vi "ListFiles.vi"() -> ()   [LabVIEW 2010]
uses:
  EDSDK-Labview.llb/kEdsStorageType.ctl
  EDSDK-Labview.llb/EdsAccess.ctl
  EDSDK-Labview.llb/kEdsTargetImageTypes.ctl
  EDSDK-Labview.llb/kEdsImageTypes.ctl
  EDSDK-Labview.llb/EdsImageQuality.ctl
  EDSDK-Labview.llb/kEdsProperties.ctl
  EDSDK-Labview.llb/kEdsImageSrcs.ctl
panel:
  out "timing details":cluster{"FileName":string, u32, "Numeric":dbl}[](array[cluster])
  in  "Image Type":T1=4 items=["Grayscale (U8)", "Grayscale (I16)", "Grayscale (SGL)", "Complex (CSG)", "RGB (U32)", "HSL (U32)", "RGB (U64)", "Grayscale (U16)"]
  out "dt":u32
  out "current file":string
  in  "full/thumbnail":bool
  in  "stop":bool
  out "Image Out":T2(plugin-control)
  out "files":T4(array[cluster]) {"format" items=["Unknown"=0, "Jpeg"=1, "CRW"=2, "RAW"=4, "CR2"=6, "MOVwithTHM"=12, "MOVwithoutTHM"=13]}
  out "subfolders":T6(array[cluster]) {"format" items=["Unknown"=0, "Jpeg"=1, "TIFF"=7, "TIFF16"=8, "RGB"=9, "RGB16"=10, "DIB"=11]}
  out "folders":T6(array[cluster]) {"format" items=["Unknown"=0, "Jpeg"=1, "TIFF"=7, "TIFF16"=8, "RGB"=9, "RGB16"=10, "DIB"=11]}
  out "disks":T9(array[cluster]) {"kEdsStorageType" items=["Non"=0, "CF"=1, "SD"=2, "HD"=4]; "EdsAccess" items=["ReadOnly"=0, "WriteOnly"=1, "ReadWrite"=2, "Error"=4294967295]}
  out "cameras":u32
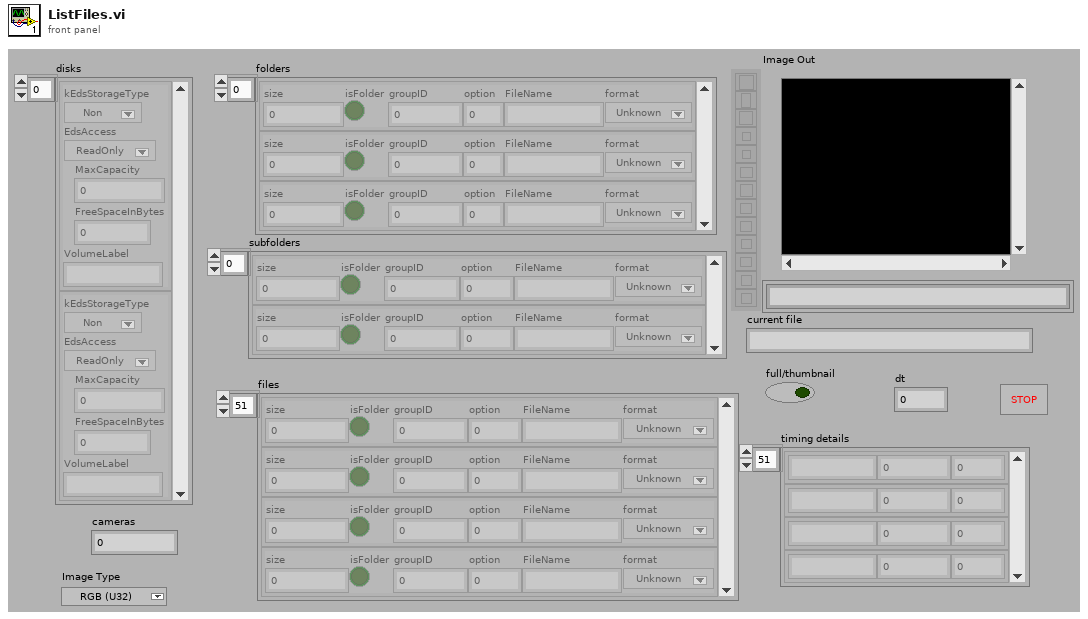
[diagram p1: front panel]
types:
  T1 = typedef "Image Type" = u32
  T2 = typedef "IMAQ Image.ctl" = refnum<image>
  T3 = typedef "kEdsImageTypes.ctl" = u32
  T4 = cluster{"size":u32, "isFolder":bool, "groupID":u32, "option":u32, "FileName":string, "format":T3}[]
  T5 = typedef "kEdsTargetImageTypes.ctl" = u32
  T6 = cluster{"size":u32, "isFolder":bool, "groupID":u32, "option":u32, "FileName":string, "format":T5}[]
  T7 = typedef "kEdsStorageType.ctl" = u32
  T8 = typedef "EdsAccess.ctl" = u32
  T9 = cluster{"kEdsStorageType":T7, "EdsAccess":T8, "MaxCapacity":u64, "FreeSpaceInBytes":u64, "VolumeLabel":string}[]
  T10 = cluster{"kEdsStorageType":T7, "EdsAccess":T8, "MaxCapacity":u64, "FreeSpaceInBytes":u64, "VolumeLabel":string}
  T11 = typedef "EdsImageQuality.ctl" = u32
  T12 = typedef "kEdsProperties.ctl" = u32
  T13 = typedef "kEdsImageSrcs.ctl" = u32
  T14 = cluster{"width":u32, "height":u32, "# components":u32, "bit depth":u32, "rect":u32[], "reserved 1":u32, "reserved 2":u32}
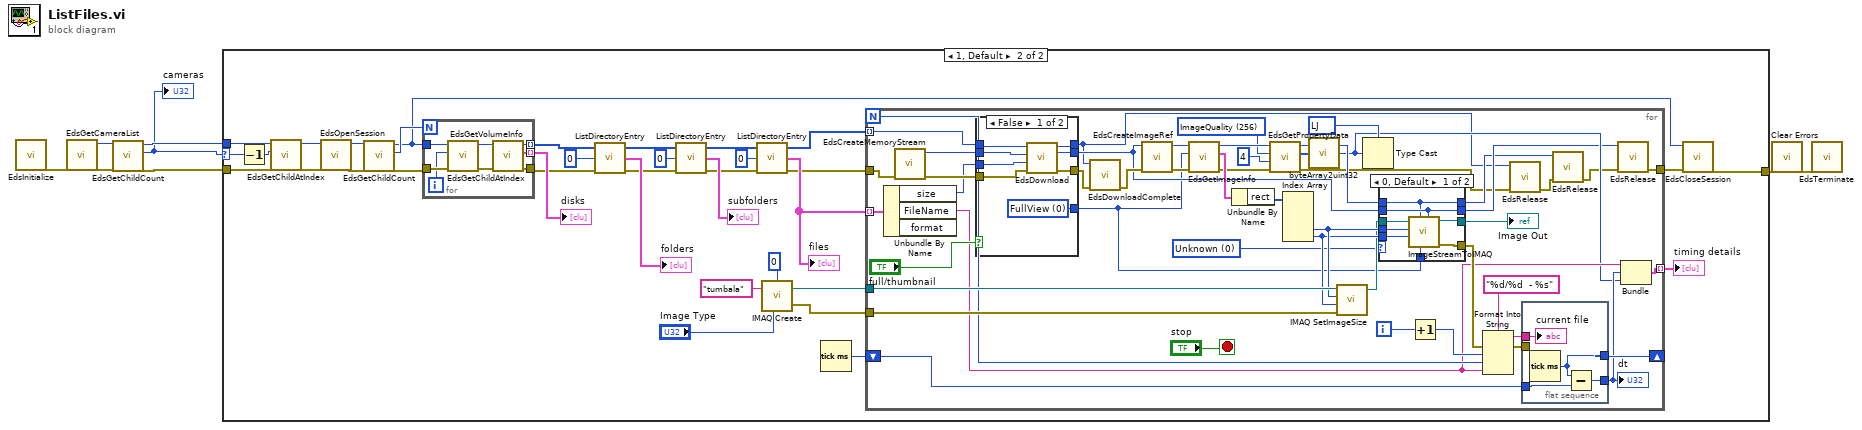
[diagram p0: block diagram]
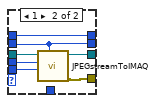
[diagram p3: hidden frame]
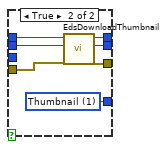
[diagram p4: hidden frame]
diagram:
  n1 = call "EdsInitialize.vi"() -> ("error out"=w8:errorcluster)  [unwired: 11 in]
  n2 = call "EdsGetCameraList.vi"("error in"=w8) -> ("error out"=w4:errorcluster, "outCameraListRef"=w5:u32)  [unwired: 9 in]
  n3 = call "EdsGetChildCount.vi"("error in"=w4, "inRef"=w5) -> ("error out"=w3:errorcluster, "count"=w1:u32, "inRef dup"=w2:u32)  [unwired: 7 in]
  "cameras" <- w1
  n4 = case shown="1, Default" w1 {
    selector: w1 -> [_ w39]
    tunnel: w2 -> [_ w41]
    tunnel: w3 -> [w9 w40]
    tunnel: [w9 w38] -> w6
    frame 0 {
    }
    frame 1, Default {
      n5 = Decrement(x=w39) -> (x-1=w44:u32)
      n6 = call "EdsGetChildAtIndex.vi"("error in"=w40, "index"=w44, "inRef"=w41) -> ("error out"=w42:errorcluster, "outRef"=w43:u32)  [unwired: 7 in]
      n7 = call "EdsOpenSession.vi"("error in"=w42, "inCameraRef"=w43) -> ("error out"=w36:errorcluster, "inCameraRef dup"=w37:u32)  [unwired: 8 in]
      n8 = call "EdsGetChildCount.vi"("error in"=w36, "inRef"=w37) -> ("error out"=w35:errorcluster, "count"=w34:u32, "inRef dup"=w33:u32)  [unwired: 7 in]
      n9 = for {
        N: w34 -> [_]
        tunnel: w33 -> [w136]
        tunnel: w35 -> [w135]
        tunnel: [w131] -> w30
        tunnel: [w130] -> w32 mode=indexing
        tunnel: [w129] -> w31 mode=indexing
        i -> [w134]
        n10 = call "EdsGetChildAtIndex.vi"("error in"=w135, "index"=w134, "inRef"=w136) -> ("error out"=w132:errorcluster, "outRef"=w133:u32)  [unwired: 7 in]
        n11 = call "EdsGetVolumeInfo.vi"("error in"=w132, "inVolumeRef"=w133) -> ("error out"=w131:errorcluster, "VolumeInfo"=w130:T10, "inVolumeRef dup"=w129:u32)  [unwired: 7 in]
      }
      "disks" <- w32
      n12 = call "ListDirectoryEntry.vi"("error out 2"=w30, "entry to descend"=0 ("index"), "Dir items at this level"=w31) -> ("error out"=w27:errorcluster, "dir List"=→"folders":T6, "inner items refs"=w26:u32[])
      n13 = call "ListDirectoryEntry.vi"("error out 2"=w27, "entry to descend"=0, "Dir items at this level"=w26) -> ("error out"=w21:errorcluster, "dir List"=→"subfolders":T6, "inner items refs"=w22:u32[])
      n14 = call "ListDirectoryEntry.vi"("error out 2"=w21, "entry to descend"=0, "Dir items at this level"=w22) -> ("error out"=w18:errorcluster, "dir List"=w19:T6, "inner items refs"=w20:u32[])
      "files" <- w19
      n15 = call "IMAQ Create"("Border Size"=0, "Image Name"="tumbala", "Image Type"="Image Type") -> ("New Image"=w13:T2, "error out"=w12:errorcluster)  [unwired: 2 in]
      n16 = Tick Count (ms)() -> (millisecond timer value=w11:u32)
      n17 = for {
        N -> [w73]
        tunnel: w20 -> [w80] mode=indexing
        tunnel: w19 -> [w81] mode=indexing
        tunnel: w18 -> [w94]
        tunnel: [w53] -> w17
        tunnel: w13 -> [w87]
        tunnel: w12 -> [w86]
        shift-right: [w69] -> _
        shift-left: w11 -> [w68]
        tunnel: [w64] -> w10 mode=indexing
        i -> [w75]
        stop <- "stop" stop-if-true
        w56 = T11 1113871 items=["LJ"=1113871, "M1J"=84999951, "M2J"=101777167, "SJ"=34668303, "LJF"=1310479, "LJN"=1244943, "MJF"=18087695, "MJN"=18022159, "SJF"=34864911, "SJN"=34799375, "S1JF"=236191503, "S1JN"=236125967, "S2JF"=252968719, "S3JF"=269745935, "LR"=6618895, "LRLJF"=6553619, "LRLJN"=6553618, "LRMJF"=6553875, "LRMJN"=6553874, "LRSJF"=6554131, "LRSJN"=6554130, "LRS1JF"=6557203, "LRS1JN"=6557202, "LRS2JF"=6557459, "LRS3JF"=6557715, "LRLJ"=6553616, "LRM1J"=6554896, "LRM2J"=6555152, "LRSJ"=6554128, "MR"=23396111, "MRLJF"=23330835, "MRLJN"=23330834, "MRMJF"=23331091, "MRMJN"=23331090, "MRSJF"=23331347, "MRSJN"=23331346, "MRS1JF"=23334419, "MRS1JN"=23334418, "MRS2JF"=23334675, "MRS3JF"=23334931, "MRLJ"=23330832, "MRM1J"=23332112, "MRM2J"=23332368, "MRSJ"=23331344, "SR"=40173327, "SRLJF"=40108051, "SRLJN"=40108050, "SRMJF"=40108307, "SRMJN"=40108306, "SRSJF"=40108563, "SRSJN"=40108562, "SRS1JF"=40111635, "SRS1JN"=40111634, "SRS2JF"=40111891, "SRS3JF"=40112147, "SRLJ"=40108048, "SRM1J"=40109328, "SRM2J"=40109584, "SRSJ"=40108560, "Unknown"=4294967295] ("EdsImageQuality")
        w57 = T12 256 items=["Unknown"=65535, "ProductName"=2, "BodyID"=3, "OwnerName"=4, "MakerName"=5, "DateTime"=6, "FirmwareVersion"=7, "BatteryLevel"=8, "CFn"=9, "SaveTo"=11, "CurrentStorage"=12, "CurrentFolder"=13, "MyMenu"=14, "BatteryQuality"=16, "HDDirectoryStructure"=32, "ImageQuality"=256, "JpegQuality"=257, "Orientation"=258, "ICCProfile"=259, "FocusInfo"=260, "DigitalExposure"=261, "WhiteBalance"=262, "ColorTemperature"=263, "WhiteBalanceShift"=264, "Contrast"=265, "ColorSaturation"=266, "ColorTone"=267, "Sharpness"=268, "ColorSpace"=269, "ToneCurve"=270, "PhotoEffect"=271, "FilterEffect"=272, "ToningEffect"=273, "ParameterSet"=274, "ColorMatrix"=275, "PictureStyle"=276, "PictureStyleDesc"=277, "ETTL2Mode"=279, "PictureStyleCaption"=512, "Linear"=768, "ClickWBPoint"=769, "WBCoeffs"=770, "GPSVersionID"=2048, "GPSLatitudeRef"=2049, "GPSLatitude"=2050, "GPSLongitudeRef"=2051, "GPSLongitude"=2052, "GPSAltitudeRef"=2053, "GPSAltitude"=2054, "GPSTimeStamp"=2055, "GPSSatellites"=2056, "GPSStatus"=2057, "GPSMapDatum"=2066, "GPSDateStamp"=2077, "AtCapture_Flag"=2147483648, "AEMode"=1024, "DriveMode"=1025, "ISOSpeed"=1026, "MeteringMode"=1027, "AFMode"=1028, "Av"=1029, "Tv"=1030, "ExposureCompensation"=1031, "FlashCompensation"=1032, "FocalLength"=1033, "AvailableShots"=1034, "Bracket"=1035, "WhiteBalanceBracket"=1036, "LensName"=1037, "AEBracket"=1038, "FEBracket"=1039, "ISOBracket"=1040, "NoiseReduction"=1041, "FlashOn"=1042, "RedEye"=1043, "FlashMode"=1044, "LensStatus"=1046, "Artist"=1048, "Copyright"=1049, "DepthOfField"=1051, "EFCompensation"=1054, "Evf_OutputDevice"=1280, "Evf_Mode"=1281, "Evf_WhiteBalance"=1282, "Evf_ColorTemperature"=1283, "Evf_DepthOfFieldPreview"=1284, "Evf_Zoom"=1287, "Evf_ZoomPosition"=1288, "Evf_FocusAid"=1289, "Evf_Histogram"=1290, "Evf_ImagePosition"=1291, "Evf_HistogramStatus"=1292, "Evf_AFMode"=1294, "Evf_CoordinateSystem"=1344, "Evf_ZoomRect"=1345] ("inPropertyID")
        w63 = T5 0 items=["Unknown"=0, "Jpeg"=1, "TIFF"=7, "TIFF16"=8, "RGB"=9, "RGB16"=10, "DIB"=11] ("format")
        n18 = Unbundle By Name(w81) -> ("size"=w82:u32, "FileName"=w66:string)  [unwired: 1 out]
        n19 = call "EdsCreateMemoryStream.vi"("error in"=w94) -> ("error out"=w93:errorcluster, "outStreamRef"=w92:u32)  [unwired: 9 in]
        n20 = case shown="False" "full/thumbnail" {
          tunnel: w80 -> [w119 w128]
          tunnel: w93 -> [w121 w127]
          tunnel: w92 -> [w116 w126]
          tunnel: [w120 w125] -> w91
          tunnel: [w118 w124] -> w46
          tunnel: [w117 w123] -> w52
          tunnel: w82 -> [w115 _]
          tunnel: [w114 w122] -> w45
          frame False {
            w114 = T13 0 items=["FullView", "Thumbnail", "Preview", "RAWThumbnail", "RAWFullView"] ("inImageSource")
            n21 = call "EdsDownload.vi"("error in"=w121, "inReadSize"=w115, "outStreamRef"=w116, "inDirItemRef"=w119) -> ("error out"=w120:errorcluster, "outStreamRef dup"=w117:u32, "inDirItemRef dup"=w118:u32)  [unwired: 5 in]
          }
          frame True {
            w122 = T13 1 items=["FullView", "Thumbnail", "Preview", "RAWThumbnail", "RAWFullView"] ("inImageSource")
            n22 = call "EdsDownloadThumbnail.vi"("error in"=w127, "outStreamRef"=w126, "inDirItemRef"=w128) -> ("error out"=w125:errorcluster, "outStreamRef dup"=w123:u32, "inDirItemRef dup"=w124:u32)  [unwired: 6 in]
          }
        }
        n23 = call "EdsDownloadComplete.vi"("error in"=w91, "inDirItemRef"=w46) -> ("error out"=w90:errorcluster)  [unwired: 9 in]
        n24 = call "EdsCreateImageRef.vi"("error in"=w90, "inStreamRef"=w52) -> ("error out"=w88:errorcluster, "outImageRef"=w89:u32)  [unwired: 8 in]
        n25 = call "EdsGetImageInfo.vi"("error in"=w88, "inImageSource"=w45, "inImageRef"=w89) -> ("error out"=w60:errorcluster, "outImageInfo"=w84:T14, "inImageRef dup"=w61:u32)  [unwired: 6 in]
        n26 = Unbundle By Name(w84) -> ("rect"=w79:u32[])
        n27 = call "EdsGetPropertyData.vi"("error in"=w60, "inPropertySize"=u32 4, "inPropertyID"=w57, "inRef"=w61) -> ("error out"=w47:errorcluster, "outPropertyData"=w55:u8[], "inRef dup"=w59:u32)  [unwired: 5 in]
        n28 = Index Array(array=w79) -> (element #3=w78:u32, element #4=w77:u32)  [unwired: 4 in, 2 out]
        n29 = call "byteArray2uint32.vi"("byteArray"=w55) -> ("uint32"=w54:u32)
        n30 = call "IMAQ SetImageSize"("error in (no error)"=w86, "Y Resolution"=w77, "X Resolution"=w78, "Image"=w87) -> ("Image Out"=w67:T2)  [unwired: 1 in, 1 out]
        n31 = Type Cast(type=w56, x=w54) -> ()  [unwired: 1 out]
        n32 = case shown="0, Default" w63 {
          tunnel: w67 -> [w100 w109]
          tunnel: [w102 w108] -> w85
          tunnel: w52 -> [w97 w104]
          tunnel: w78 -> [w99 w107]
          tunnel: w77 -> [w98 w106]
          tunnel: [w101 w105] -> w70
          tunnel: w59 -> [w96 w103]
          tunnel: [w97 w104] -> w51
          tunnel: [w96 w103] -> w49
          tunnel: w45 -> [w95 _]
          frame 0, Default {
            n33 = call "ImageStreamToIMAQ.vi"("inStreamRef"=w97, "inImageRef"=w96, "inImageSource (Thumbnail for evf)"=w95, "height"=w98, "width"=w99, "Image"=w100) -> ("error out"=w101:errorcluster, "Image Out"=w102:T2)  [unwired: 4 in]
          }
          frame 1 {
            n34 = call "JPEGstreamToIMAQ.vi"("inStream"=w104, "height"=w106, "width"=w107, "Image"=w109) -> ("error out"=w105:errorcluster, "Image Out"=w108:T2)  [unwired: 3 in]
          }
        }
        "Image Out" <- w85
        n35 = Increment(x=w75) -> (x+1=w74:i32)
        n36 = Format Into String(format string="%d/%d  - %s", error in=w70, w74, w73, w66) -> (resulting string=w71:string, error out=w62:errorcluster)  [unwired: 1 in]
        n37 = call "EdsRelease.vi"("error in"=w47, "inRef"=w46) -> ("error out"=w48:errorcluster)  [unwired: 7 in, 2 out]
        n38 = flat-sequence {
          tunnel: w71 -> [w113]
          tunnel: [w112] -> w69
          tunnel: w68 -> [w111]
          tunnel: [w110] -> w65
          tunnel: w62 -> [_]
          frame #0 {
            n39 = Tick Count (ms)() -> (millisecond timer value=w112:u32)
            n40 = Subtract(x=w112, y=w111) -> (x-y=w110:u32)
            "current file" <- w113
          }
        }
        n41 = call "EdsRelease.vi"("error in"=w48, "inRef"=w49) -> ("error out"=w50:errorcluster)  [unwired: 7 in, 2 out]
        n42 = call "EdsRelease.vi"("error in"=w50, "inRef"=w51) -> ("error out"=w53:errorcluster)  [unwired: 7 in, 2 out]
        n43 = Bundle("FileName"=w66, w65, "uint32"=w54) -> (w64:cluster{"FileName":string, u32, "uint32":u32})  [unwired: 1 in]
        "dt" <- w65
      }
      "timing details" <- w10
      n44 = call "EdsCloseSession.vi"("error in"=w17, "inCameraRef"=w33) -> ("error out"=w38:errorcluster)  [unwired: 8 in, 1 out]
    }
  }
  n45 = call <vilib>:"Clear Errors.vi"("error in (no error)"=w6) -> ("error out"=w7:errorcluster)  [unwired: 6 in]
  n46 = call "EdsTerminate.vi"("error in"=w7) -> ()  [unwired: 10 in, 1 out]
